vi "Diagnostics File Path.vi"() -> (0 "diagnostics file path":path)   [LabVIEW 2021, in "Diagnostics.lvlib"]
uses:
  Diagnostics.lvlib
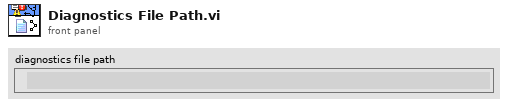
[diagram p1: front panel]
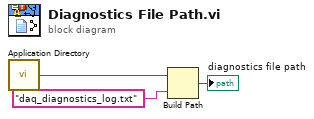
[diagram p0: block diagram]
diagram:
  n1 = call <vilib>:"Application Directory.vi"() -> ("Application Directory"=w1:path)
  n2 = Build Path(base path=w1, name or relative path="daq_diagnostics_log.txt") -> (appended path=→"diagnostics file path":path)
